vi "GetSequenceIndicesTable.vi"(8 "error in (no error)":errorcluster, 11 "VariableManagerRef in":refnum<vi>) -> (0 "error out":errorcluster, 2 "SequenceIndicesTable":string[][](array[string]), 3 "VariableManagerRef out":refnum<vi>)   [LabVIEW 2013, in "VariableManagerAPI.lvlib"]
doc: "Return an array of string representing all sequence index definitions in the variable manager.\n\nSequenceIndexName | Steps"
uses:
  VariableManagerAPI.lvlib
  VariableManager/VariableManager.lvclass
  SequenceIndex/SequenceIndex.lvclass
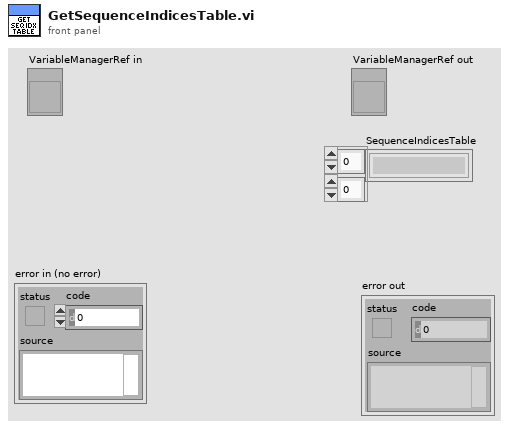
[diagram p1: front panel]
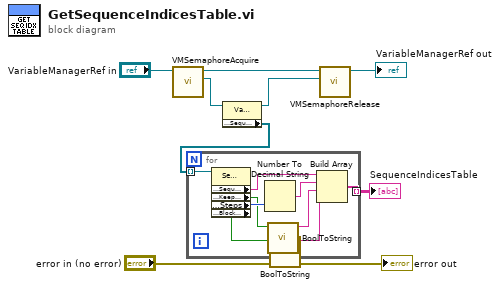
[diagram p0: block diagram]
diagram:
  n1 = call "VMSemaphoreAcquire.vi"("VariableManagerRef in"="VariableManagerRef in") -> ("VariableManager"=w3:refnum<class "VariableManager.lvclass">, "VariableManagerRef out"=w6:refnum<vi>)  [unwired: 7 in, 2 out]
  n2 = property class="VariableManager.lvclass"(reference=w3) -> (reference out=w2:refnum<class "VariableManager.lvclass">, "Accessors:SequenceIndices"=w4:refnum<class "SequenceIndex.lvclass">[])  [unwired: 1 in, 1 out]
  n3 = for {
    tunnel: w4 -> [w17] mode=indexing
    tunnel: [w15] -> w1 mode=indexing
    n4 = property class="SequenceIndex.lvclass"(reference=w17) -> ("Accessors:SequenceIndexName"=w16:string, "Accessors:Keep Linear on Random"=w12:bool, "Accessors:Steps"=w14:u32, "Accessors:Block Randomize"=w10:bool)  [unwired: 1 in, 2 out]
    n5 = Number To Decimal String(number=w14) -> (decimal integer string=w13:string)  [unwired: 1 in]
    n6 = call "BoolToString.vi"("BooleanIn"=w12) -> ("String"=w11:string)  [unwired: 10 in]
    n7 = call "BoolToString.vi"("BooleanIn"=w10) -> ("String"=w9:string)  [unwired: 10 in]
    n8 = Build Array(w16, w13, w11, w9) -> (w15:string[])
  }
  "SequenceIndicesTable" <- w1
  n9 = call "VMSemaphoreRelease.vi"("VariableManager"=w2, "VariableManagerRef in"=w6) -> ("VariableManagerRef out"=→"VariableManagerRef out":refnum<vi>)  [unwired: 8 in, 1 out]
  "error out" <- "error in (no error)"
